vi "Start Sync.vi"(8 "error in (no error)":errorcluster, 10 "current time":timestamp, 11 "gRPC Server in":refnum<class "HVC4.lvclass">) -> (0 "error out":errorcluster, 3 "gRPC Server out":refnum<class "HVC4.lvclass">)   [LabVIEW 2019, in "HVC4.lvlib" / "HVC4.lvclass"]
uses:
  HVC4.lvclass
  RPC Messages/measurementservice_DMMConfigRequest/measurementservice_DMMConfigRequest_Data.ctl
  RPC Messages/measurementservice_SMUConfigRequest/measurementservice_SMUConfigRequest_Data.ctl
  HVC4.lvclass/HVC4.ctl
  RPC Messages/measurementservice_QueryResponse/measurementservice_QueryResponse_Data.ctl
  RPC Messages/measurementservice_DMMConfigResponse/measurementservice_DMMConfigResponse_Data.ctl
  RPC Messages/measurementservice_ErrorOut/measurementservice_ErrorOut_Data.ctl
  RPC Messages/measurementservice_DMMVoltageData/measurementservice_DMMVoltageData_Data.ctl
  RPC Messages/measurementservice_SMUConfigResponse/measurementservice_SMUConfigResponse_Data.ctl
  RPC Messages/measurementservice_SMUCurrentData/measurementservice_SMUCurrentData_Data.ctl
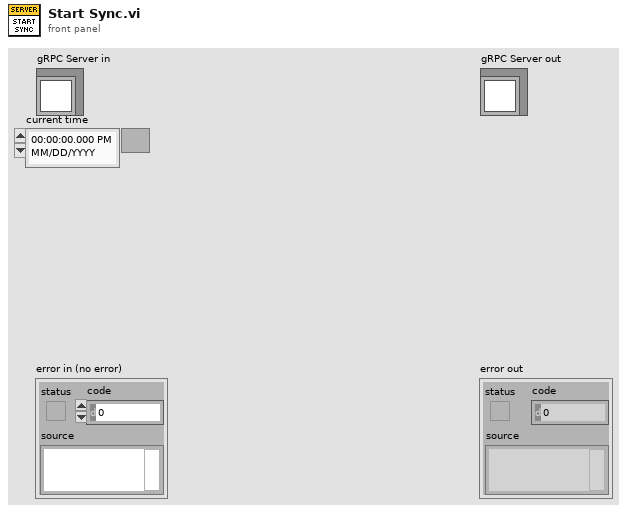
[diagram p1: front panel]
types:
  T1 = typedef "HVC4.lvlib/HVC4.lvclass/measurementservice_DMMConfigRequest_Data.ctl" = cluster{"DMMName":string, "DMMFunction":i32, "DMMResolution":sgl, "DMMRange":sgl, "DMMSampleCount":i32, "DMMApertureTimeUnit":i32, "DMMApertureTime":sgl, "DMMNumberofAverages":i32, "DMMAutoZero":i32, "DMMADCCalibration":i32, "DMMSettleTime":sgl}
  T2 = typedef "HVC4.lvlib/HVC4.lvclass/measurementservice_SMUConfigRequest_Data.ctl" = cluster{"SMUName":string, "SMUChannels":i32, "SMUSourceMode":i32, "SMUOutputFunction":i32, "SMUSourceTransientResponse":i32, "SMUCurrent":sgl, "SMUCurrentLevelRange":sgl, "SMUMeasurementSense":i32, "SMUMeasurementApertureTime":sgl, "SMUSourceAdvancedSourceDelay":sgl, "SMUVoltage":sgl, "SMUMeasurementAdvancedDCNoiseRejection":i32}
  T3 = cluster{"measurementservice_DMMConfigRequest_Data":T1, "measurementservice_SMUConfigRequest_Data":T2}
  T4 = typedef "HVC4.lvlib/HVC4.lvclass/measurementservice_QueryResponse_Data.ctl" = cluster{"message":string, "status":i32}
  T5 = typedef "HVC4.lvlib/HVC4.lvclass/measurementservice_ErrorOut_Data.ctl" = cluster{"errCode":i32, "errMessage":string}
  T6 = typedef "HVC4.lvlib/HVC4.lvclass/measurementservice_DMMConfigResponse_Data.ctl" = cluster{"DMMName":string, "DMMFunction":i32, "DMMResolution":sgl, "DMMRange":sgl, "DMMSampleCount":i32, "DMMApertureTimeUnit":i32, "DMMApertureTime":sgl, "DMMNumberofAverages":i32, "DMMAutoZero":i32, "DMMADCCalibration":i32, "DMMSettleTime":sgl, "error":T5}
  T7 = typedef "HVC4.lvlib/HVC4.lvclass/measurementservice_DMMVoltageData_Data.ctl" = cluster{"voltage":sgl[], "error":T5}
  T8 = typedef "HVC4.lvlib/HVC4.lvclass/measurementservice_SMUConfigResponse_Data.ctl" = cluster{"SMUName":string, "SMUChannels":i32, "SMUSourceMode":i32, "SMUOutputFunction":i32, "SMUSourceTransientResponse":i32, "SMUCurrent":sgl, "SMUCurrentLevelRange":sgl, "SMUMeasurementSense":i32, "SMUMeasurementApertureTime":sgl, "SMUSourceAdvancedSourceDelay":sgl, "SMUVoltage":sgl, "SMUMeasurementAdvancedDCNoiseRejection":i32, "error":T5}
  T9 = typedef "HVC4.lvlib/HVC4.lvclass/measurementservice_SMUCurrentData_Data.ctl" = cluster{"current":sgl, "error":T5}
  T10 = typedef "HVC4.lvlib/HVC4.lvclass/Server gRPC UEs.ctl" = cluster{"Invoke gRPC UE":refnum<user-event>, "Query gRPC UE":refnum<user-event>, "Register gRPC UE":refnum<user-event>, "ConfigureDMM gRPC UE":refnum<user-event>, "PerformDMMVoltageMeasurement gRPC UE":refnum<user-event>, "ConfigureSMU gRPC UE":refnum<user-event>, "EnableSMUOutput gRPC UE":refnum<user-event>, "DisableSMUOutput gRPC UE":refnum<user-event>, "PerformSMUCurrentMeasurement gRPC UE":refnum<user-event>}
  T11 = typedef "HVC4.lvlib/gprc-lvsupport.lvlib/grpcId.ctl" = u64
  T12 = typedef "HVC4.lvlib/HVC4.lvclass/measurementservice_QueryRequest_Data.ctl" = cluster{"query":string}
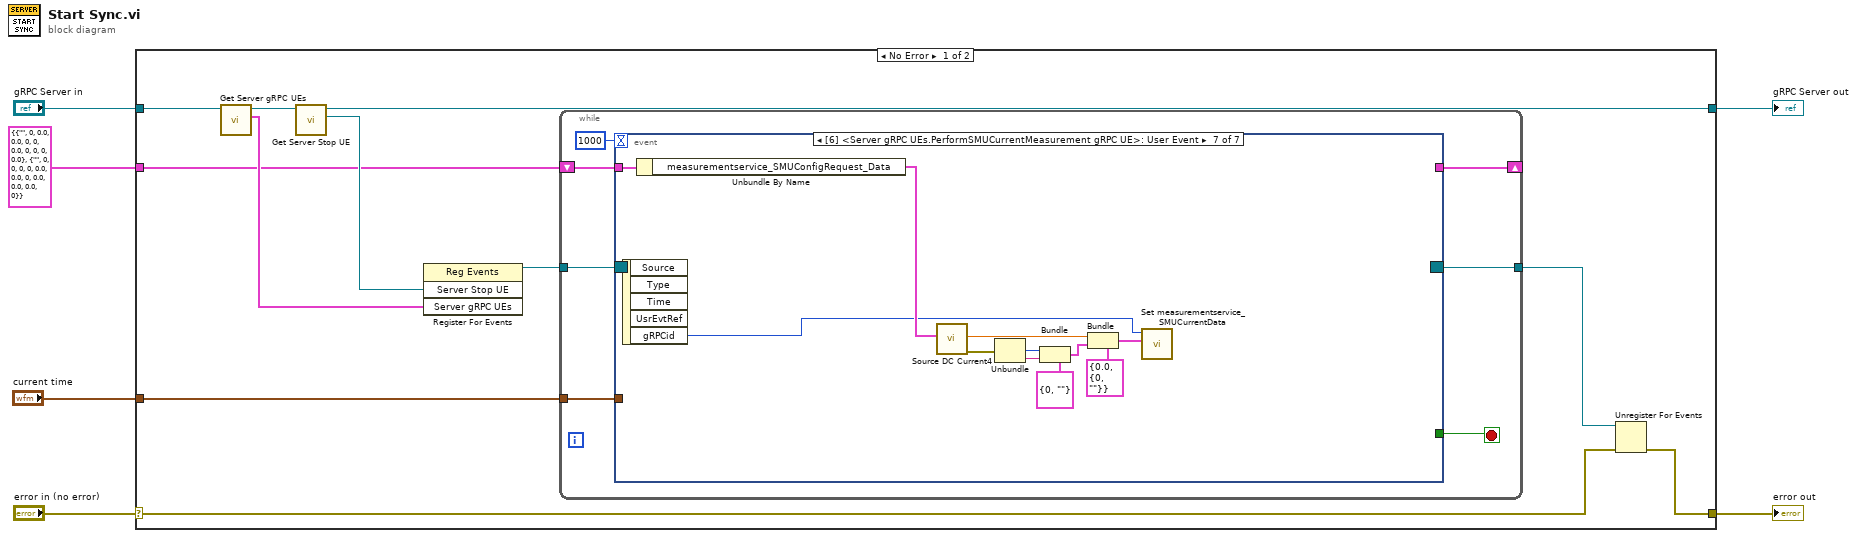
[diagram p0: block diagram]
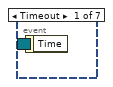
[diagram p2: hidden frame]
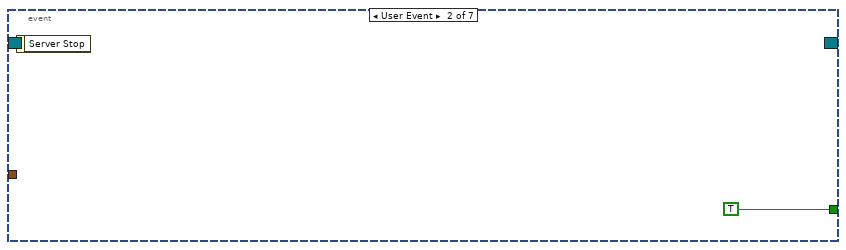
[diagram p3: hidden frame]
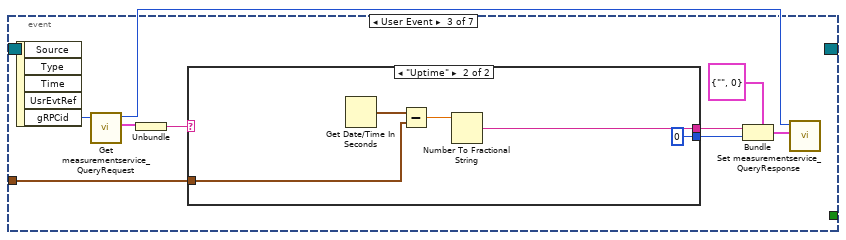
[diagram p4: hidden frame]
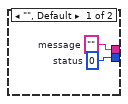
[diagram p5: hidden frame]
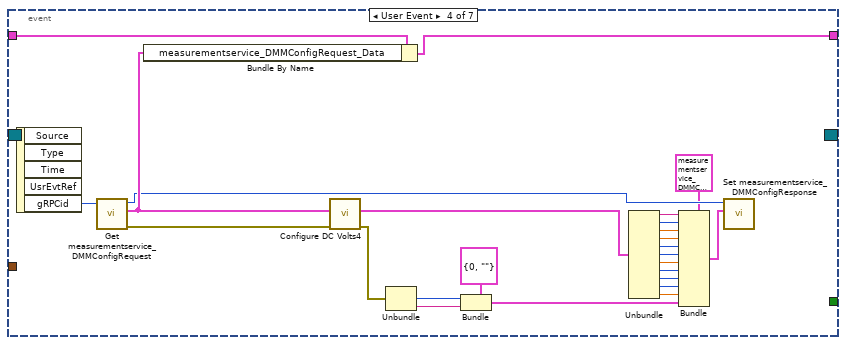
[diagram p6: hidden frame]
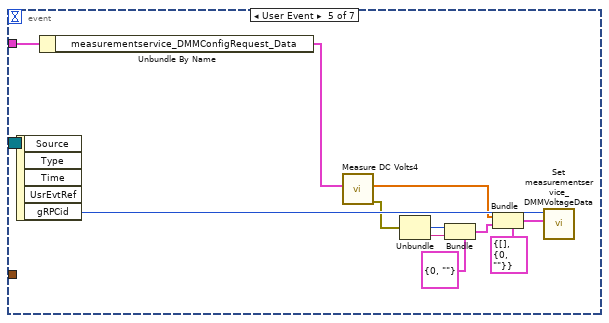
[diagram p7: hidden frame]
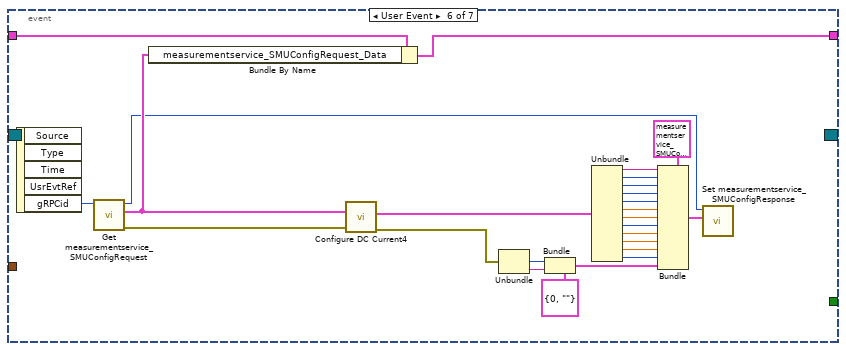
[diagram p8: hidden frame]
diagram:
  n1 = case shown="No Error" "error in (no error)" {
    selector: "error in (no error)" -> [w10 w116]
    tunnel: [w9 w116] -> w5
    tunnel: [w13 w115] -> w3
    tunnel: "gRPC Server in" -> [w17 w115]
    tunnel: "current time" -> [w8 _]
    tunnel: T3 {"measurementservice_DMMConfigRequest_Data"={"DMMName"="", "DMMFunction"=0, "DMMResolution"=0.0, "DMMRange"=0.0, "DMMSampleCount"=0, "DMMApertureTimeUnit"=0, "DMMApertureTime"=0.0, "DMMNumberofAverages"=0, "DMMAutoZero"=0, "DMMADCCalibration"=0, "DMMSettleTime"=0.0}, "measurementservice_SMUConfigRequest_Data"={"SMUName"="", "SMUChannels"=0, "SMUSourceMode"=0, "SMUOutputFunction"=0, "SMUSourceTransientResponse"=0, "SMUCurrent"=0.0, "SMUCurrentLevelRange"=0.0, "SMUMeasurementSense"=0, "SMUMeasurementApertureTime"=0.0, "SMUSourceAdvancedSourceDelay"=0.0, "SMUVoltage"=0.0, "SMUMeasurementAdvancedDCNoiseRejection"=0}} -> [w7 _]
    frame No Error {
      n2 = call "Get Server gRPC UEs.vi"("OOP Server in"=w17) -> ("Server gRPC UEs"=w14:T10, "OOP Server out"=w16:refnum<class "HVC4.lvclass">)  [unwired: 9 in]
      n3 = call "Get Server Stop UE.vi"("OOP Server in"=w16) -> ("Server Stop UE"=w15:refnum<user-event>, "OOP Server out"=w13:refnum<class "HVC4.lvclass">)  [unwired: 9 in]
      n4 = register-events(w15, w14) -> (reference out=w12:refnum<event-registration>)  [unwired: 2 in, 1 out]
      n5 = while {
        tunnel: w12 -> [w24]
        tunnel: [w22] -> w11
        tunnel: w8 -> [w20]
        shift-right: [w18] -> _
        shift-left: w7 -> [w19]
        stop <- w23 stop-if-true
        n6 = event "RPC Methods Event Structure" shown="[6] <Server gRPC UEs.PerformSMUCurrentMeasurement gRPC UE>: User Event" {
          selector: w24 -> [_ _ _ _ _ _ _]
          dyn-events: [_ _ _ _ _ _ _] -> w22
          timeout: 1000 -> [_ _ _ _ _ _ _]
          tunnel: [_ TRUE _ _ _ _ _] -> w23
          tunnel: w20 -> [_ _ w31 _ _ _ _]
          tunnel: w19 -> [_ _ _ w65 w74 w102 w112]
          tunnel: [_ _ _ w64 _ w101 _] -> w18
          event Timeout {
            n7 = event-data() -> ()  [unwired: 1 in, 1 out]
          }
          event User Event {
            n8 = event-data() -> ()  [unwired: 1 in, 1 out]
          }
          event User Event {
            n9 = event-data() -> ("gRPCid"=w30:T11)  [unwired: 1 in, 4 out]
            n10 = call "Get measurementservice_QueryRequest.vi"("gRPCid"=w30) -> ("Message Data"=w29:T12, "gRPCid out"=w28:T11)  [unwired: 8 in, 1 out]
            n11 = Unbundle(w29) -> ("query"=w34:string)
            n12 = case shown="\"Uptime\"" w34 {
              tunnel: [w36 0 ("status")] -> w33
              tunnel: [w35 w39] -> w32
              tunnel: w31 -> [_ w37]
              frame "", Default {
                w35 = ""  # message
                w36 = 0  # status
              }
              frame "Uptime" {
                n13 = Get Date/Time In Seconds() -> (seconds since 1Jan1904=w41:timestamp)
                n14 = Subtract(x=w41, y=w37) -> (x-y=w40:dbl)
                n15 = Number To Fractional String(number=w40) -> (F-format string=w39:string)  [unwired: 3 in]
              }
            }
            n16 = Bundle(cluster=T4 {"message"="", "status"=0} ("measurementservice_QueryResponse_Data"), "message"=w32, "status"=w33) -> (w27:T4)
            n17 = call "Set measurementservice_QueryResponse.vi"("Message Data"=w27, "gRPCid"=w28) -> ()  [unwired: 9 in, 1 out]
          }
          event User Event {
            n18 = event-data() -> ("gRPCid"=w66:T11)  [unwired: 1 in, 4 out]
            n19 = call "Get measurementservice_DMMConfigRequest.vi"("gRPCid"=w66) -> ("error out"=w42:errorcluster, "Message Data"=w63:T1, "gRPCid out"=w62:T11)  [unwired: 8 in]
            n20 = Bundle By Name(cluster=w65, "measurementservice_DMMConfigRequest_Data"=w63) -> (w64:T3)
            n21 = call "Configure DC Volts4.vi"("error in (no error)"=w42, "measurementservice_DMMConfigRequest_Data"=w63) -> ("error out"=w47:errorcluster, "measurementservice_DMMConfigRequest_Data Out"=w59:T1)  [unwired: 8 in]
            n22 = Unbundle(w47) -> ("code"=w45:i32, "source"=w44:string)  [unwired: 1 out]
            n23 = Bundle(cluster=T5 {"errCode"=0, "errMessage"=""} ("error"), "errCode"=w45, "errMessage"=w44) -> (w43:T5)
            n24 = Unbundle(w59) -> ("DMMName"=w58:string, "DMMFunction"=w57:i32, "DMMResolution"=w56:sgl, "DMMRange"=w55:sgl, "DMMSampleCount"=w54:i32, "DMMApertureTimeUnit"=w53:i32, "DMMApertureTime"=w52:sgl, "DMMNumberofAverages"=w51:i32, "DMMAutoZero"=w50:i32, "DMMADCCalibration"=w49:i32, "DMMSettleTime"=w48:sgl)
            n25 = Bundle(cluster=T6 {"DMMName"="", "DMMFunction"=0, "DMMResolution"=0.0, "DMMRange"=0.0, "DMMSampleCount"=0, "DMMApertureTimeUnit"=0, "DMMApertureTime"=0.0, "DMMNumberofAverages"=0, "DMMAutoZero"=0, "DMMADCCalibration"=0, "DMMSettleTime"=0.0, "error"={"errCode"=0, "errMessage"=""}} ("measurementservice_DMMConfigResponse_Data"), "DMMName"=w58, "DMMFunction"=w57, "DMMResolution"=w56, "DMMRange"=w55, "DMMSampleCount"=w54, "DMMApertureTimeUnit"=w53, "DMMApertureTime"=w52, "DMMNumberofAverages"=w51, "DMMAutoZero"=w50, "DMMADCCalibration"=w49, "DMMSettleTime"=w48, "error"=w43) -> (w60:T6)
            n26 = call "Set measurementservice_DMMConfigResponse.vi"("Message Data"=w60, "gRPCid"=w62) -> ()  [unwired: 9 in, 1 out]
          }
          event User Event {
            n27 = event-data() -> ("gRPCid"=w75:T11)  [unwired: 1 in, 4 out]
            n28 = Unbundle By Name(w74) -> ("measurementservice_DMMConfigRequest_Data"=w73:T1)
            n29 = call "Measure DC Volts4.vi"("measurementservice_DMMConfigRequest_Data"=w73) -> ("error out"=w71:errorcluster, "Measurement Array (Volts)"=w72:dbl[])  [unwired: 9 in]
            n30 = Unbundle(w71) -> ("code"=w68:i32, "source"=w67:string)  [unwired: 1 out]
            n31 = Bundle(cluster=T5 {"errCode"=0, "errMessage"=""} ("error"), "errCode"=w68, "errMessage"=w67) -> (w69:T5)
            n32 = Bundle(cluster=T7 {"voltage"=[], "error"={"errCode"=0, "errMessage"=""}} ("measurementservice_DMMVoltageData_Data"), "voltage"=w72, "error"=w69) -> (w76:T7)
            n33 = call "Set measurementservice_DMMVoltageData.vi"("Message Data"=w76, "gRPCid"=w75) -> ()  [unwired: 9 in, 1 out]
          }
          event User Event {
            n34 = event-data() -> ("gRPCid"=w103:T11)  [unwired: 1 in, 4 out]
            n35 = call "Get measurementservice_SMUConfigRequest.vi"("gRPCid"=w103) -> ("error out"=w84:errorcluster, "Message Data"=w98:T2, "gRPCid out"=w78:T11)  [unwired: 8 in]
            n36 = Bundle By Name(cluster=w102, "measurementservice_SMUConfigRequest_Data"=w98) -> (w101:T3)
            n37 = call "Configure DC Current4.vi"("error in (no error)"=w84, "measurementservice_SMUConfigRequest_Data"=w98) -> ("error out"=w83:errorcluster, "measurementservice_SMUConfigRequest_Data Out"=w97:T2)  [unwired: 8 in]
            n38 = Unbundle(w83) -> ("code"=w81:i32, "source"=w80:string)  [unwired: 1 out]
            n39 = Bundle(cluster=T5 {"errCode"=0, "errMessage"=""} ("error"), "errCode"=w81, "errMessage"=w80) -> (w79:T5)
            n40 = Unbundle(w97) -> ("SMUName"=w96:string, "SMUChannels"=w95:i32, "SMUSourceMode"=w94:i32, "SMUOutputFunction"=w93:i32, "SMUSourceTransientResponse"=w92:i32, "SMUCurrent"=w91:sgl, "SMUCurrentLevelRange"=w90:sgl, "SMUMeasurementSense"=w89:i32, "SMUMeasurementApertureTime"=w88:sgl, "SMUSourceAdvancedSourceDelay"=w87:sgl, "SMUVoltage"=w86:sgl, "SMUMeasurementAdvancedDCNoiseRejection"=w85:i32)
            n41 = Bundle(cluster=T8 {"SMUName"="", "SMUChannels"=0, "SMUSourceMode"=0, "SMUOutputFunction"=0, "SMUSourceTransientResponse"=0, "SMUCurrent"=0.0, "SMUCurrentLevelRange"=0.0, "SMUMeasurementSense"=0, "SMUMeasurementApertureTime"=0.0, "SMUSourceAdvancedSourceDelay"=0.0, "SMUVoltage"=0.0, "SMUMeasurementAdvancedDCNoiseRejection"=0, "error"={"errCode"=0, "errMessage"=""}} ("measurementservice_SMUConfigResponse_Data"), "SMUName"=w96, "SMUChannels"=w95, "SMUSourceMode"=w94, "SMUOutputFunction"=w93, "SMUSourceTransientResponse"=w92, "SMUCurrent"=w91, "SMUCurrentLevelRange"=w90, "SMUMeasurementSense"=w89, "SMUMeasurementApertureTime"=w88, "SMUSourceAdvancedSourceDelay"=w87, "SMUVoltage"=w86, "SMUMeasurementAdvancedDCNoiseRejection"=w85, "error"=w79) -> (w99:T8)
            n42 = call "Set measurementservice_SMUConfigResponse.vi"("Message Data"=w99, "gRPCid"=w78) -> ()  [unwired: 9 in, 1 out]
          }
          event User Event {
            n43 = event-data() -> ("gRPCid"=w105:T11)  [unwired: 1 in, 4 out]
            n44 = Unbundle By Name(w112) -> ("measurementservice_SMUConfigRequest_Data"=w111:T2)
            n45 = call "Source DC Current4.vi"("measurementservice_SMUConfigRequest_Data"=w111) -> ("error out"=w110:errorcluster, "Current Measurement"=w108:sgl)  [unwired: 7 in, 2 out]
            n46 = Unbundle(w110) -> ("code"=w114:i32, "source"=w113:string)  [unwired: 1 out]
            n47 = Bundle(cluster=T5 {"errCode"=0, "errMessage"=""} ("error"), "errCode"=w114, "errMessage"=w113) -> (w106:T5)
            n48 = Bundle(cluster=T9 {"current"=0.0, "error"={"errCode"=0, "errMessage"=""}} ("measurementservice_SMUCurrentData_Data"), "current"=w108, "error"=w106) -> (w104:T9)
            n49 = call "Set measurementservice_SMUCurrentData.vi"("Message Data"=w104, "gRPCid"=w105) -> ()  [unwired: 9 in, 1 out]
          }
        }
      }
      n50 = Unregister For Events(event registration refnum=w11, error in=w10) -> (error out=w9:errorcluster)
    }
    frame Error {
    }
  }
  "error out" <- w5
  "gRPC Server out" <- w3
